vi "BlinkingLED_Main.vi"() -> ()   [LabVIEW 2014]
uses:
  <vilib>/MakerHub/LINX/Public/Peripherals/Digital/Digital Write 1 Chan.vi
  <vilib>/MakerHub/LINX/Public/Peripherals/Digital/Digital Write N Chans.vi
  <vilib>/MakerHub/LINX/Private/Local IO/LinxDigitalWrite.vi
  <vilib>/MakerHub/LINX/Public/Utilities/Check Channel.vi
  <vilib>/MakerHub/LINX/Private/Local IO/Handle Errors.vi
  <vilib>/MakerHub/LINX/Public/Utilities/Open Local.vi
  <vilib>/MakerHub/LINX/Private/Utilties/Generate Error.vi
  LedState_class/LedState.lvclass
  <vilib>/MakerHub/LINX/LMH-LINX.lvlib
panel:
  out "Error Out":errorcluster
  out "LED":bool
  in  "Stop":bool
  # "Blinking LED on Pin 7 (GPIO 4)"
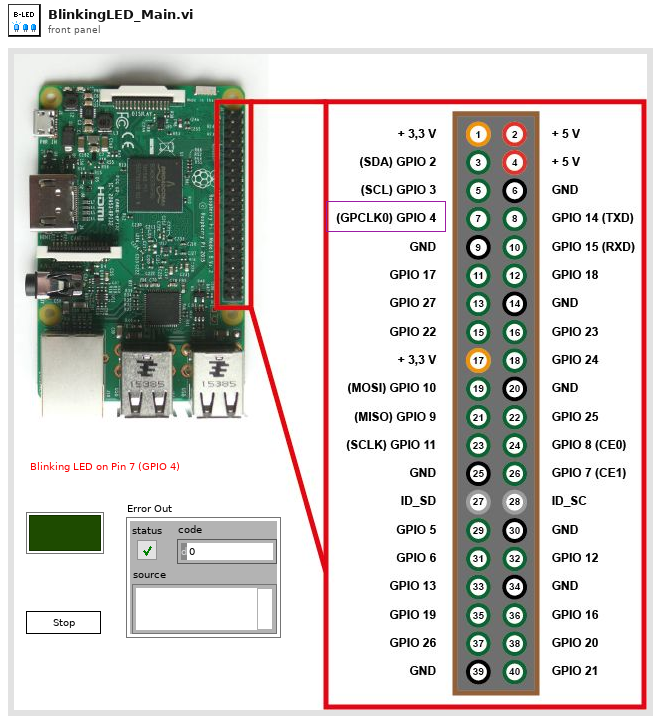
[diagram p1: front panel]
types:
  T1 = typedef "LMH-LINX.lvlib/LINX Ref.ctl" = cluster{"IO":T2, "Interface":T3, "LINX Device Config":T4}
  T2 = typedef "LMH-LINX.lvlib/Platform.ctl" = enum16{"Remote", "Local"}
  T3 = typedef "LMH-LINX.lvlib/Interface.ctl" = enum16{"Serial", "TCP"}
  T4 = typedef "LMH-LINX.lvlib/Device.lvlib/LINX Device Config.ctl" = cluster{"Interface":T3, "COM Port":refnum<visa-resource-name>, "TCP Configuration":T5, "Device Family":u8, "Device ID":u8, "Device Name":string, "TCP Ref":refnum<k5>, "Channels":T6}
  T5 = typedef "LMH-LINX.lvlib/Device.lvlib/TCP Config.ctl" = cluster{"IP Address":string, "Port":u16}
  T6 = typedef "LMH-LINX.lvlib/Channels.ctl" = cluster{"DI":u8[], "DO":u8[], "AI":u8[], "AO":u8[], "PWM":u8[], "QE":u8[], "UART":u8[], "I2C 2":u8[], "SPI":u8[], "CAN":u8[], "Servo":u8[], "AI Ref (V)":dbl, "AI Resolution (Bits)":u8, "AO Ref (V)":dbl, "AO Resolution (Bits)":u8}
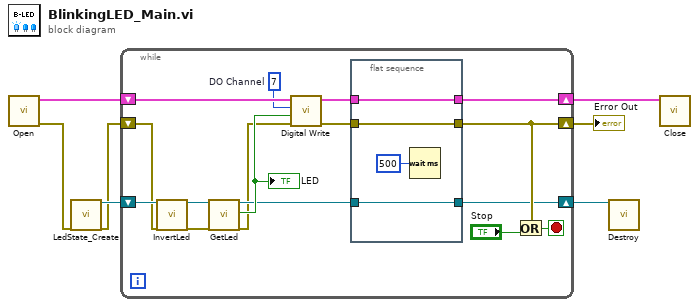
[diagram p0: block diagram]
diagram:
  n1 = call-poly <vilib>:"Open.vi"() -> ("Error Out"=w2:errorcluster, "LINX Resource"=w7:T1)  [unwired: 9 in, 1 out]
  n2 = call "LedState_Create.vi"("error in (no error)"=w2) -> ("reference out"=w4:refnum<class "LedState.lvclass">, "error out"=w1:errorcluster)  [unwired: 17 in]
  n3 = while {
    shift-right: [w16] -> w6
    shift-left: w7 -> [w18]
    shift-right: [w21] -> w5
    shift-left: w1 -> [w9]
    shift-right: [w20] -> w3
    shift-left: w4 -> [w14]
    stop <- w22 stop-if-true
    w15 = u8 7  # DO Channel
    n4 = call-dynamic "InvertLed.vi"("reference in"=w14, "error in (no error)"=w9) -> ("reference out"=w13:refnum<class "LedState.lvclass">, "error out"=w10:errorcluster)  [unwired: 16 in]
    n5 = call-dynamic "GetLed.vi"("reference in"=w13, "error in (no error)"=w10) -> ("reference out"=w11:refnum<class "LedState.lvclass">, "Led"=w12:bool, "error out"=w8:errorcluster)  [unwired: 15 in]
    "LED" <- w12
    n6 = call-poly <vilib>:"Digital Write.vi"("Error In"=w8, "Output Value"=w12, "DO Channel"=w15, "LINX Resource"=w18) -> ("Error Out"=w19:errorcluster, "LINX Resource"=w17:T1)  [unwired: 6 in]
    n7 = flat-sequence {
      tunnel: [w24] -> w21
      tunnel: w19 -> [w24]
      tunnel: w11 -> [w27]
      tunnel: [w27] -> w20
      tunnel: w17 -> [w25]
      tunnel: [w25] -> w16
      frame #0 {
        n8 = Wait (ms)(milliseconds to wait=u32 500) -> ()  [unwired: 1 out]
      }
    }
    n9 = Or(x=w21, y="Stop") -> (x .or. y?=w22:bool)
  }
  "Error Out" <- w5
  n10 = call-dynamic "Destroy.vi"("reference in"=w3) -> ()  [unwired: 17 in, 2 out]
  n11 = call <vilib>:"Close.vi"("LINX Resource"=w6) -> ()  [unwired: 10 in, 1 out]
